vi "PH_ImageCoG_Plotter.constructor.vi"(0 "name":string, 2 "data in":string, 5 "error in":errorcluster) -> (14 "i ref out":refnum<vi>, 16 "data out":string, 19 "error out":errorcluster)   [LabVIEW 2014, in "PH_ImageCoG_Plotter.lvlib"]
doc: "This class is forseen to operate on an image: it calculates several beam profile values. This class is connected to the class PH_ImageCalibrator which has to be used to produce a background image, and to the class PH_IEEE1394Camera to get an image from.\n\nThis class is part of the PHELIX user layer.\n\nauthor: Stefan Götte, GSI\n\nLicense Agreement for this software:\n\nCopyright (C)\nGesellschaft für Schwerionenforschung, GSI\nPlanckstr. 1\n64291 Darmstadt\nGermany\n\nContact: D.Beck@gsi.de \n\nThis program is free software; you can redistribute it and/or modify it under the terms of the \nGNU General Public License as published by the Free Software Foundation; either version 2 of \nthe license, or (at your option) any later version.\n\nThis program is distributed in the hope that it will be useful, but WITHOUT ANY WARRANTY; \nwithout even the implied warranty of MERCHANTABILITY or FITNESS FOR A PARTICULAR PURPOSE. See the GNU General License for more details (http://www.gnu.org).\n\nGesellschaft für Schwerionenforschung, GSI\nPlanckstr. 1, 64291 Darmstadt, Germany\nFor all questions and ideas contact: M.Richter@gsi.de, H.Brand@gsi.de or D.Beck@gsi.de.\nLast update: 16-JUN-2004"
uses:
  PH_ImageCoG_Plotter.lvlib
  CS_Core/BaseProcess/BaseProcess.lvlib
  PH_Basics/PH_Img_BaseClass/PH_Img_BaseClass.lvlib
  PH_Basics/PH_Class/PH_Class.lvlib
  CS_Core/CSObj/CSObj.lvlib
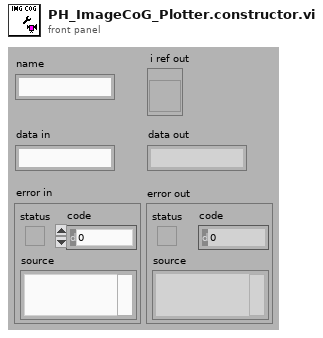
[diagram p1: front panel]
types:
  T1 = enum16{"SetAttribute", "GetAttribute", "CreateAttribute", "DestroyAttribute", "DestroyAllAtributes"}
  T2 = typedef "PH_ImageCoG_Plotter.lvlib/PH_ImageCoG_Plotter.i attribute.ctl" = cluster{"GUI Refs":cluster{"Delete":refnum<vi>, "Calibration status":refnum<vi>, "BI subtracted":refnum<vi>, "calc Beam Anal":refnum<vi>, "CoG - x":refnum<vi>, "CoG - y":refnum<vi>, "Type":refnum<vi>, "Center":refnum<vi>, "exp - X":refnum<vi>, "exp - Y":refnum<vi>, "Delta - X":refnum<vi>, "Delta - Y":refnum<vi>, "Available Cams":refnum<vi>, "CoG X":refnum<vi>, "CoG Y":refnum<vi>, "Delta X":refnum<vi>, "Delta Y":refnum<vi>, "Export Data":refnum<vi>, "Calibration data":refnum<vi>}, "Calibration":cluster{"Status":T3, "Calibration data":T4, "Calibration Data File":path}, "Beam Analysis":cluster{"on":bool, "exp - X":i32, "exp - Y":i32, "Type":bool, "Data":cluster{"current time":timestamp, "CoG-x":dbl, "CoG-y":dbl, "Delta-x":dbl, "Delta-y":dbl}[], "Datasets strored":i32, "Dataarray Size":i32}, "Cam instances":string[], "DIM Service Events":T5[], "Images":cluster{"Background":T8, "OP":T8, "GUI":T8}}
  T3 = typedef "PH_StatusHandler.lvlib/PH_StatusHandler.Status.ctl" = i16
  T4 = typedef "PH_ImageCalibrator.lvlib/PH_ImageCalibrator.Calibration Data.ctl" = cluster{"Date":string, "Time":string, "Cam Settings":cluster{"Cam ID":string, "Gain":dbl, "Brightness":dbl, "Shutter":dbl, "Cam Error":bool, "Mode":i32}, "Background Image":cluster{"Image":dbl[][], "Image Error":bool}, "Linear Calibration":cluster{"Calibration Factor":dbl, "not mm or mrad":bool}, "Energy Calibration":cluster{"Calibration Factor":dbl, "no mJ":bool}}
  T5 = typedef "BaseProcess.lvlib/BaseProcess.event definition.ctl" = cluster{"CAEEvtDef":T6, "Data Descriptor":T7}
  T6 = typedef "CAEObj.lvlib/CAEObj.event definition.ctl" = cluster{"URL":string, "enable":bool, "ignoreResID":bool}
  T7 = typedef "BaseProcess.lvlib/BaseProcess.descriptor string definition.ctl" = string
  T8 = typedef "IMAQ Image.ctl" = refnum<image>
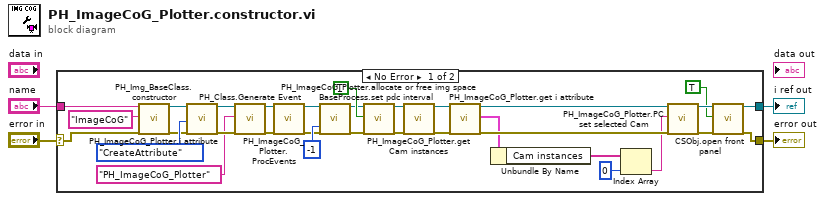
[diagram p0: block diagram]
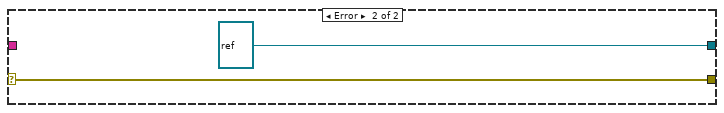
[diagram p2: hidden frame]
diagram:
  n1 = case shown="No Error" "error in" {
    selector: "error in" -> [w23 w37]
    tunnel: [w8 refnum<vi> refnum ("i ref out")] -> w4
    tunnel: [w6 w37] -> w3
    tunnel: "name" -> [w33 _]
    frame No Error {
      n2 = call "PH_Img_BaseClass.constructor.vi"("name"=w33, "data in"="ImageCoG" ("DB entry"), "error in(no error)"=w23) -> ("i ref out"=w32:refnum<vi>, "error out"=w31:errorcluster)  [unwired: 14 in, 1 out]
      n3 = call "PH_ImageCoG_Plotter.i attribute.vi"("VI Refnum"=w32, "Action"=T1."CreateAttribute", "error in (no error)"=w31) -> ("VI Refnum out"=w29:refnum<vi>, "error out"=w30:errorcluster)  [unwired: 14 in, 1 out]
      n4 = call "PH_Class.Generate Event.vi"("i ref in"=w29, "Class"="PH_ImageCoG_Plotter", "error in (no error)"=w30) -> ("i ref out"=w27:refnum<vi>, "error out"=w26:errorcluster)  [unwired: 15 in]
      n5 = call "PH_ImageCoG_Plotter.ProcEvents.vi"("i ref in"=w27, "error in"=w26) -> ("i ref out"=w25:refnum<vi>, "error out"=w24:errorcluster)  [unwired: 16 in]
      n6 = call "BaseProcess.set pdc interval.vi"("i ref in"=w25, "PeriodicInterval [ms]"=-1 ("PeriodicInterval"), "error in (no error)"=w24) -> ("i ref out"=w11:refnum<vi>, "error out"=w10:errorcluster)  [unwired: 14 in, 1 out]
      n7 = call "PH_ImageCoG_Plotter.allocate or free img space.vi"("i ref in"=w11, "Allocate?"=TRUE, "error in (no error)"=w10) -> ("i ref out"=w12:refnum<vi>, "error out"=w13:errorcluster)  [unwired: 15 in]
      n8 = call "PH_ImageCoG_Plotter.get Cam instances.vi"("i ref in"=w12, "error in"=w13) -> ("i ref out"=w15:refnum<vi>, "error out"=w14:errorcluster)  [unwired: 16 in]
      n9 = call "PH_ImageCoG_Plotter.get i attribute.vi"("i ref in"=w15, "error in (no error)"=w14) -> ("i ref out"=w16:refnum<vi>, "i attribute"=w20:T2, "error out"=w21:errorcluster)  [unwired: 15 in]
      n10 = Unbundle By Name(w20) -> ("Cam instances"=w19:string[])
      n11 = Index Array(array=w19, index=0) -> (element=w17:string)
      n12 = call "PH_ImageCoG_Plotter.PC set selected Cam.vi"("VI in"=w16, "Camera to select"=w17, "error in (no error)"=w21) -> ("VI out"=w9:refnum<vi>, "error out"=w7:errorcluster)  [unwired: 15 in]
      n13 = call "CSObj.open front panel.vi"("i ref in"=w9, "frontPanelOpen"=TRUE ("front panel open"), "error in (no error)"=w7) -> ("i ref out"=w8:refnum<vi>, "error out"=w6:errorcluster)  [unwired: 15 in]
    }
    frame Error {
    }
  }
  "i ref out" <- w4
  "error out" <- w3
